vi "Attach Debugger.vi"(8 "error in (no error)":errorcluster, 11 "Process In":refnum<class "Process.lvclass">) -> (0 "error out":errorcluster)   [LabVIEW 2020]
uses:
  <vilib>/Astemes/Triarc Framework/Process/Process.lvclass
  <vilib>/Astemes/Triarc Framework/Process/Process.lvclass/Process.ctl
  <vilib>/Utility/error.llb/Clear Errors.vi
  <vilib>/Utility/error.llb/Error Cluster From Error Code.vi
  <vilib>/ErrorRing/Error Ring.xnode
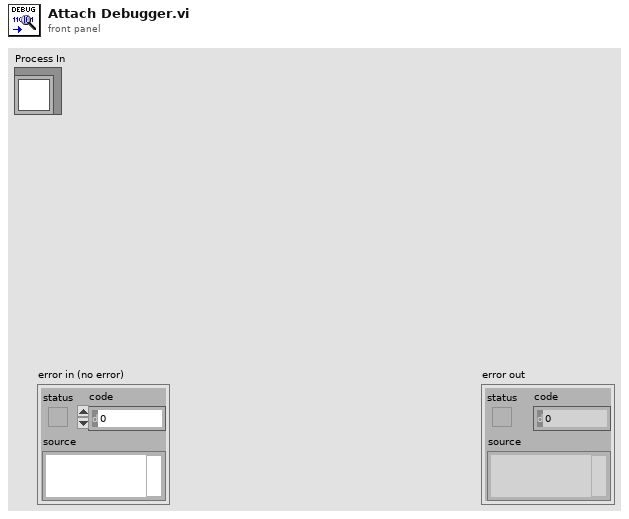
[diagram p1: front panel]
types:
  T1 = typedef "TF.lvlib/Process.lvclass/Lifecycle State.ctl" = enum16{"Uninitialized", "Initialized", "Started", "Running", "Stopped", "Finished"}
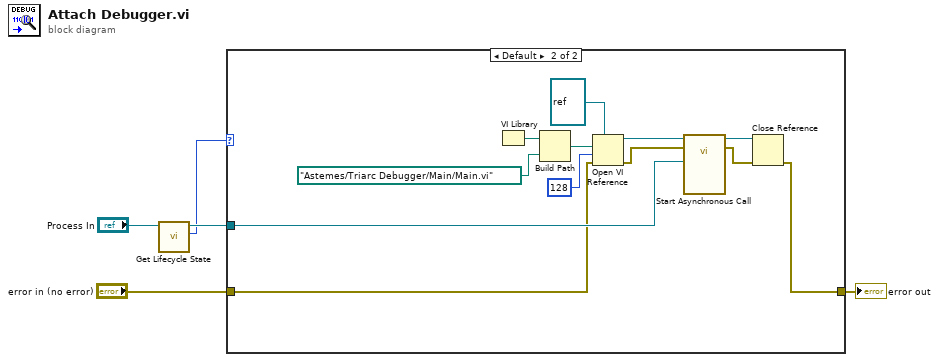
[diagram p0: block diagram]
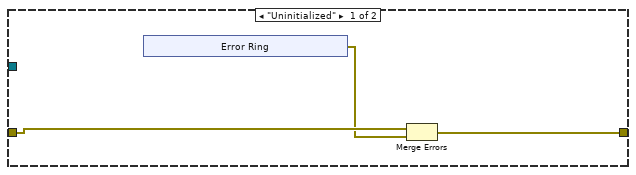
[diagram p2: hidden frame]
diagram:
  n1 = call <vilib>:"Get Lifecycle State.vi"("Process In"="Process In") -> ("Lifecycle State"=w1:T1, "Process Out"=w2:refnum<class "Process.lvclass">)  [unwired: 7 in, 2 out]
  n2 = case shown="Default" w1 {
    tunnel: [w7 w19] -> w4
    tunnel: "error in (no error)" -> [w8 w17]
    tunnel: w2 -> [_ w18]
    frame "Uninitialized" {
      n3 = xnode "Error Ring"() -> ("error out"=w6:errorcluster)
      n4 = Merge Errors(w8, w6) -> (w7:errorcluster)
    }
    frame Default {
      n5 = VI Library() -> (path=w15:path)
      n6 = Build Path(base path=w15, name or relative path=path "Astemes/Triarc Debugger/Main/Main.vi") -> (appended path=w13:path)
      n7 = Open VI Reference(type specifier VI Refnum (for type only)=refnum<vi> refnum, vi path=w13, options=128, error in (no error)=w17) -> (vi reference=w23:refnum<vi>, error out=w22:errorcluster)  [unwired: 2 in]
      n8 = call-by-ref "Start Asynchronous Call"(reference=w23, error in=w22, "Top Level Process In"=w18) -> (reference out=w20:refnum<vi>, error out=w21:errorcluster)  [unwired: 11 in]
      n9 = Close Reference(reference=w20, error in (no error)=w21) -> (error out=w19:errorcluster)
    }
  }
  "error out" <- w4
